vi "Analyse_string_array.vi"(0 "String array":string[](array[string])) -> (1 "Unique strings":string[](array[string]), 2 "Frequency":i32[](array[numeric]))   [LabVIEW 2022 SP3]
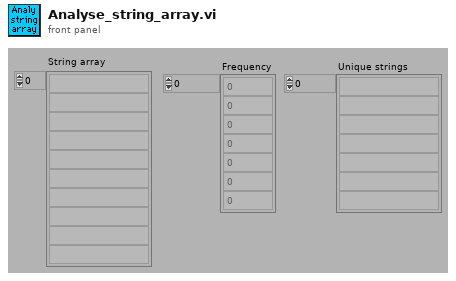
[diagram p1: front panel]
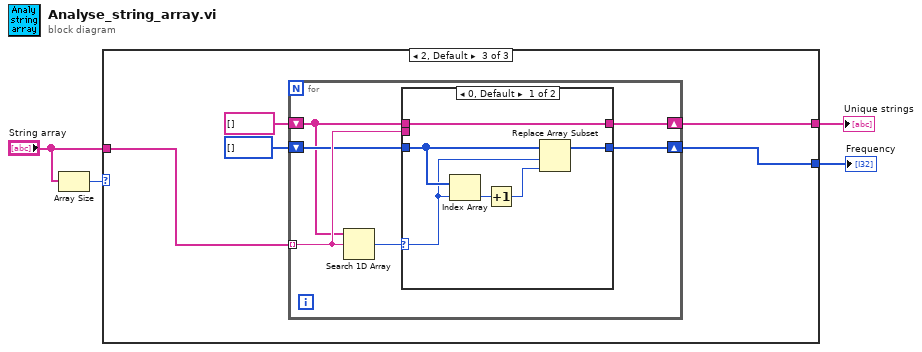
[diagram p0: block diagram]
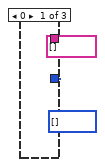
[diagram p2: hidden frame]
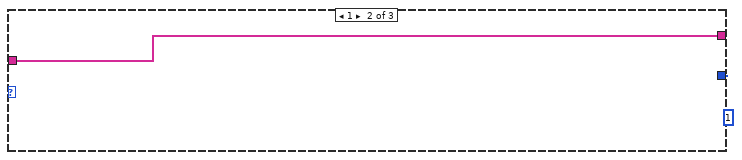
[diagram p3: hidden frame]
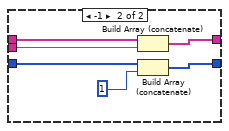
[diagram p4: hidden frame]
diagram:
  n1 = Array Size(array="String array") -> (size(s)=w3:i32)
  n2 = case shown="2, Default" w3 {
    tunnel: [i32[] [] w7 w12] -> w1
    tunnel: "String array" -> [_ w9 w14]
    tunnel: [string[] [] w9 w13] -> w2
    frame 0 {
    }
    frame 1 {
      n3 = Build Array(1) -> (w7:i32[])
    }
    frame 2, Default {
      n4 = for {
        shift-right: [w19] -> w13
        shift-left: string[] [] -> [w15]
        shift-right: [w17] -> w12
        shift-left: i32[] [] -> [w18]
        tunnel: w14 -> [w20] mode=indexing
        n5 = Search 1D Array(1D array=w15, element=w20) -> (index of element=w16:i32)  [unwired: 1 out]
        n6 = case shown="0, Default" w16 {
          selector: w16 -> [w21 _]
          tunnel: w15 -> [w26 w32]
          tunnel: w20 -> [_ w31]
          tunnel: [w26 w30] -> w19
          tunnel: w18 -> [w23 w29]
          tunnel: [w22 w28] -> w17
          frame 0, Default {
            n7 = Index Array(array=w23, index=w21) -> (element=w25:i32)
            n8 = Increment(x=w25) -> (x+1=w24:i32)
            n9 = Replace Array Subset(array=w23, new element=w24, index=w21) -> (w22:i32[])
          }
          frame -1 {
            n10 = Build Array (concatenate)(w32, w31) -> (w30:string[])
            n11 = Build Array (concatenate)(w29, 1) -> (w28:i32[])
          }
        }
      }
    }
  }
  "Frequency" <- w1
  "Unique strings" <- w2
